vi "wait_on_initialization.vi"(10 "milliseconds_to_wait(1000)":u32=1000, 11 "state":u16) -> ()   [LabVIEW 2020]
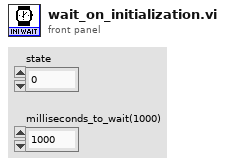
[diagram p1: front panel]
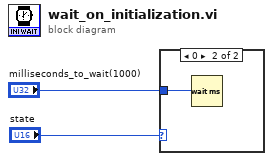
[diagram p0: block diagram]
diagram:
  n1 = case shown="0" "state" {
    tunnel: "milliseconds_to_wait(1000)" -> [_ w3]
    frame Default {
    }
    frame 0 {
      n2 = Wait (ms)(milliseconds to wait=w3) -> ()  [unwired: 1 out]
    }
  }
